vi "Convert Tree Tag to OD index.vi"(6 "subindex format":string="%04xsub%02x", 7 "index format":string="%04x", 8 "error in":errorcluster, 11 "Tag":string) -> (0 "error out":errorcluster, 3 "index":cluster{u16, u8, u8})   [LabVIEW 2013]
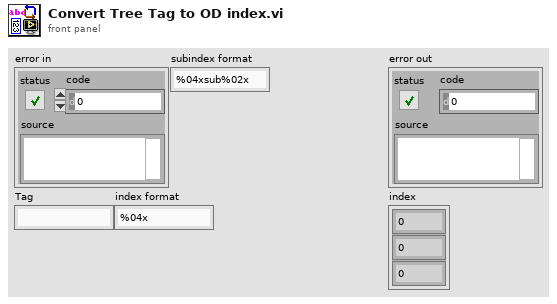
[diagram p1: front panel]
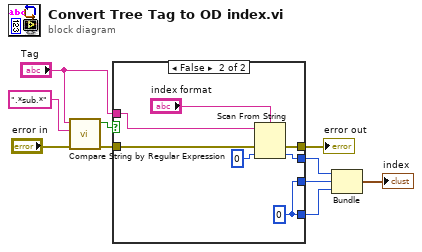
[diagram p0: block diagram]
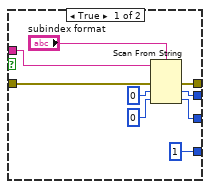
[diagram p2: hidden frame]
diagram:
  n1 = call "Compare String by Regular Expression.vi"("error in"="error in", "regular expression"=".*sub.*", "String"="Tag") -> ("error out"=w2:errorcluster, "x = y?"=w1:bool)  [unwired: 7 in]
  n2 = case shown="False" w1 {
    tunnel: "Tag" -> [w18 w23]
    tunnel: w2 -> [w17 w26]
    tunnel: [w16 w25] -> w10
    tunnel: [w13 w21] -> w9
    tunnel: [w12 w20] -> w8
    tunnel: [u8 1 w20] -> w7
    frame True {
      n3 = Scan From String(format string="subindex format", input string=w18, error in=w17, default 1=u16 0, default 2=u8 0) -> (error out=w16:errorcluster, output 1=w13:u16, output 2=w12:u8)  [unwired: 1 in, 2 out]
    }
    frame False {
      w20 = u8 0
      n4 = Scan From String(format string="index format", input string=w23, error in=w26, default 1=u16 0) -> (error out=w25:errorcluster, output 1=w21:u16)  [unwired: 1 in, 2 out]
    }
  }
  "error out" <- w10
  n5 = Bundle(w9, w8, w7) -> (→"index":cluster{u16, u8, u8})  [unwired: 1 in]
